vi "Student t CDF.vi"(10 "k degrees of freedom":i32=1, 11 "x":dbl=1.0) -> (0 "error":i32, 2 "1-cdf(x)":dbl=0.2500000000000001 format="%.6g", 3 "cdf(x)":dbl=0.7499999999999999 format="%.6g")   [LabVIEW 2020, in "NI_Gmath.lvlib"]
doc: "Computes the continuous cumulative distribution function (CDF), or the probability that the random variate X, where X describes the selected distribution type, has a value less than or equal to <B>x</B>. You must manually select the polymorphic instance to use."
uses:
  NI_Gmath.lvlib
  st_error_code.ctl
panel:
  # "Student t CDF"
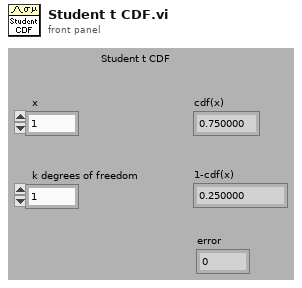
[diagram p1: front panel]
types:
  T1 = typedef "NI_Gmath.lvlib/st_error_code.ctl" = i32
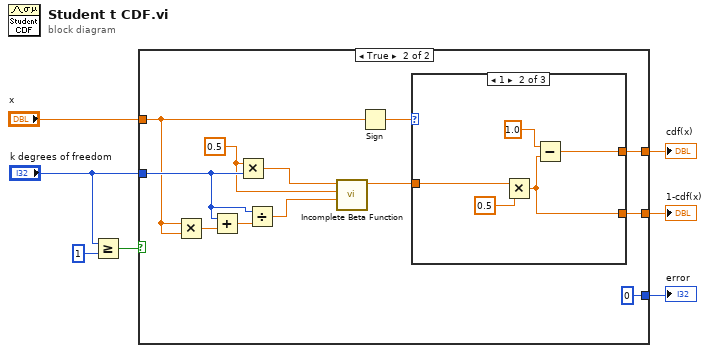
[diagram p0: block diagram]
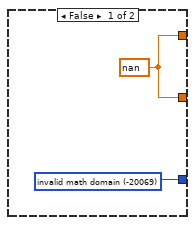
[diagram p2: hidden frame]
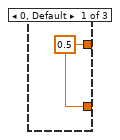
[diagram p3: hidden frame]
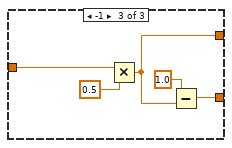
[diagram p4: hidden frame]
diagram:
  n1 = Greater Or Equal?(x="k degrees of freedom", y=1) -> (x >= y?=w5:bool)
  n2 = case shown="True" w5 {
    tunnel: [w8 0 ("invalid math domain")] -> w7
    tunnel: [w9 w13] -> w4
    tunnel: "x" -> [_ w19]
    tunnel: "k degrees of freedom" -> [_ w20]
    tunnel: [w9 w12] -> w3
    frame False {
      w8 = T1 -20069 items=["invalid math domain"=-20069, "Fourier interpolation size m >= n"=-20070, "empty array"=-20003] ("stat interp error code")
      w9 = nan
    }
    frame True {
      w17 = 0.5 ("x")
      n3 = Multiply(x=w19, y=w19) -> (x*y=w16:dbl)
      n4 = Add(x=w20, y=w16) -> (x+y=w15:dbl)
      n5 = Multiply(x=w17, y=w20) -> (x*y=w18:dbl)
      n6 = Divide(x=w20, y=w15) -> (x/y=w10:dbl)
      n7 = call "Incomplete Beta Function.vi"("a"=w10, "y"=w17, "x"=w18) -> ("b(x, y, a)"=w11:dbl)  [unwired: 8 in]
      n8 = Sign(1:w19) -> (0:w14:dbl)
      n9 = case shown="1" w14 {
        tunnel: [w22 w24 w29] -> w13
        tunnel: w11 -> [_ w26 w32]
        tunnel: [w22 w23 w28] -> w12
        frame 0, Default {
          w22 = 0.5 ("x")
        }
        frame 1 {
          n10 = Multiply(x=w26, y=0.5 ("x")) -> (x*y=w23:dbl)
          n11 = Subtract(x=1.0, y=w23) -> (x-y=w24:dbl)
        }
        frame -1 {
          n12 = Multiply(x=w32, y=0.5 ("x")) -> (x*y=w29:dbl)
          n13 = Subtract(x=1.0, y=w29) -> (x-y=w28:dbl)
        }
      }
    }
  }
  "cdf(x)" <- w4
  "error" <- w7
  "1-cdf(x)" <- w3
